vi "Get array details.vi"(8 "error in (no error)":errorcluster, 10 "Current obejct":variant, 11 "Separate object string":string) -> (0 "error out":errorcluster, 1 "Required object":string, 2 "Non-index array?":bool, 3 "Is array?":bool, 4 "Array contained cluster?":bool, 5 "Complete Array?":bool)   [LabVIEW 2015]
uses:
  <vilib>/Utility/Data Type/Type Definitions/Data Type.ctl
  <vilib>/regexp/Match Regular Expression.xnode
  <vilib>/Utility/Data Type/NI_Data Type.lvlib
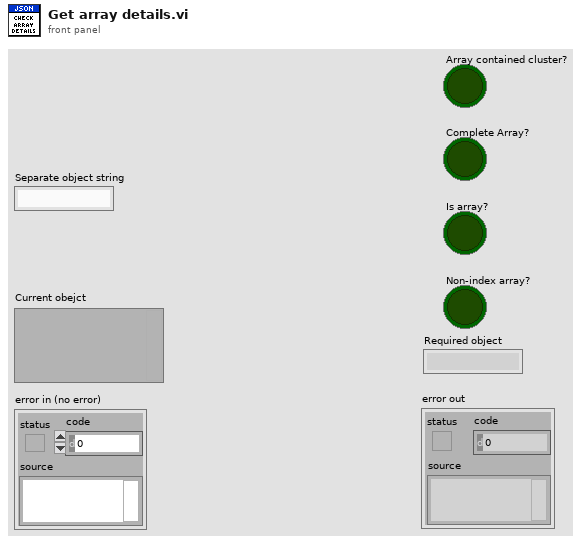
[diagram p1: front panel]
types:
  T1 = typedef "NI_Data Type.lvlib/Data Type.ctl" = enum8{"Invalid Type", "Void", "I8", "I16", "I32", "I64", "U8", "U16", "U32", "U64", "Single Float", "Double Float", "Extended Float", "Single Complex", "Double Complex", "Extended Complex", "Enum U8", "Enum U16", "Enum U32", "Enum U64", "Single Float With Unit", "Double Float With Unit", "Extended Float With Unit", "Single Complex with Unit", "Double Complex with Unit", "Extended Complex with Unit", "Boolean", "String", "Path", "Picture", "Tag", "Array", "Cluster", "Variant", "LV Variant", "Waveform", "Timestamp", "Digital Waveform", "Digital Data", "ExpressData", "Refnum", "External Data", "VI", "Poly VI", "LabVIEW Class Instance", "Fixed Point"}
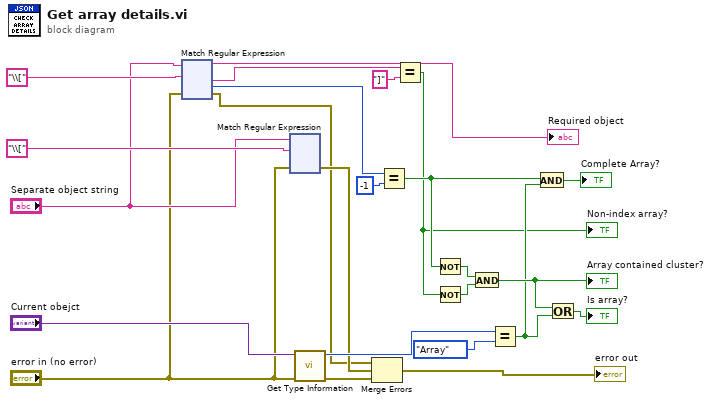
[diagram p0: block diagram]
diagram:
  n1 = xnode "Match Regular Expression"("input string"="Separate object string", "regular expression"="\\[", "error in"="error in (no error)") -> ("before match"=→"Required object":string, "after match"=w15:string, "offset past match"=w9:i32, "error out"=w11:errorcluster)  [unwired: 3 in, 1 out]
  n2 = xnode "Match Regular Expression"("input string"="Separate object string", "regular expression"="\\[", "error in"="error in (no error)") -> ("error out"=w19:errorcluster)  [unwired: 3 in, 4 out]
  n3 = call <vilib>:"Get Type Information.vi"("error in (no error)"="error in (no error)", "Variant"="Current obejct") -> ("error out"=w18:errorcluster, "Type"=w23:T1)  [unwired: 5 in, 3 out]
  n4 = Merge Errors(w11, w19, w18) -> (→"error out":errorcluster)
  n5 = Equal?(x=w9, y=-1) -> (x = y?=w7:bool)
  n6 = Equal?(x=w15, y="]") -> (x = y?=w1:bool)
  "Non-index array?" <- w1
  n7 = Not(x=w7) -> (.not. x?=w6:bool)
  n8 = Not(x=w1) -> (.not. x?=w5:bool)
  n9 = And(x=w6, y=w5) -> (x .and. y?=w4:bool)
  "Array contained cluster?" <- w4
  n10 = Equal?(x=w23, y=Data_Type."Array") -> (x = y?=w3:bool)
  n11 = And(x=w7, y=w3) -> (x .and. y?=→"Complete Array?":bool)
  n12 = Or(x=w4, y=w3) -> (x .or. y?=→"Is array?":bool)
